vi "Execute.vi"(8 "error in":errorcluster, 11 "Change Speaker Position in":refnum<class "Change Speaker Position.lvclass">) -> (0 "error out":errorcluster, 1 "Next Step?":bool, 2 "MSG":string, 3 "Change Speaker Position out":refnum<class "Change Speaker Position.lvclass">)   [LabVIEW 2015, in "Change Speaker Position.lvclass"]
uses:
  Change Speaker Position.lvclass
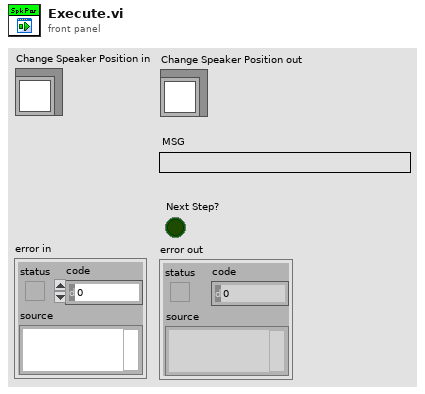
[diagram p1: front panel]
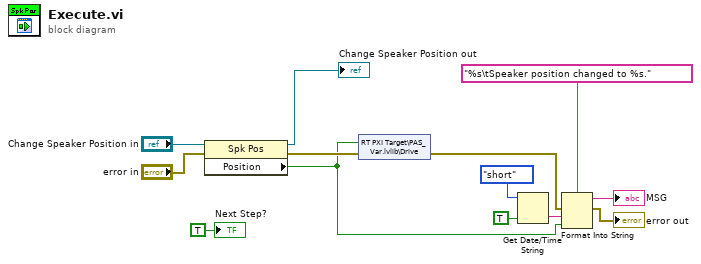
[diagram p0: block diagram]
diagram:
  n1 = property class="Spk Pos"(reference="Change Speaker Position in", error in="error in") -> (reference out=→"Change Speaker Position out":refnum<class "Change Speaker Position.lvclass">, error out=w3:errorcluster, "Position"=w1:bool)
  n2 = shared-variable "RT PXI Target\\PAS_Var.lvlib\\Drive"(w1, error in=w3) -> (error out=w2:errorcluster)
  n3 = Get Date/Time String(date format (0)=enum16{"short", "long", "abbreviated"}."short", want seconds? (F)=TRUE) -> (time string=w11:string)  [unwired: 1 in, 1 out]
  n4 = Format Into String(format string="%s\tSpeaker position changed to %s.", error in=w2, w11, w1) -> (resulting string=→"MSG":string, error out=→"error out":errorcluster)  [unwired: 1 in]
  "Next Step?" <- TRUE ("Next Step?")
